vi "Create Report subVI.vi"(8 "error in (no error)":errorcluster) -> (0 "error out":errorcluster, 3 "new file path (Not A Path if cancelled)":path)   [LabVIEW 2016]
uses:
  <vilib>/Utility/sysdir.llb/System Directory Type.ctl
  <vilib>/Utility/file.llb/Write Delimited Spreadsheet (DBL).vi
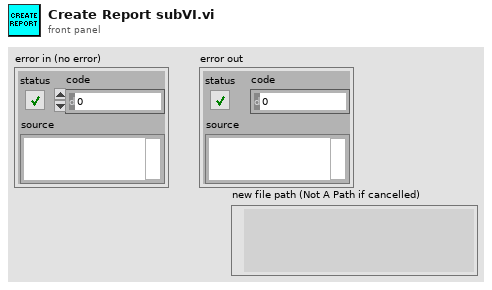
[diagram p1: front panel]
types:
  T1 = typedef "System Directory Type.ctl" = i32
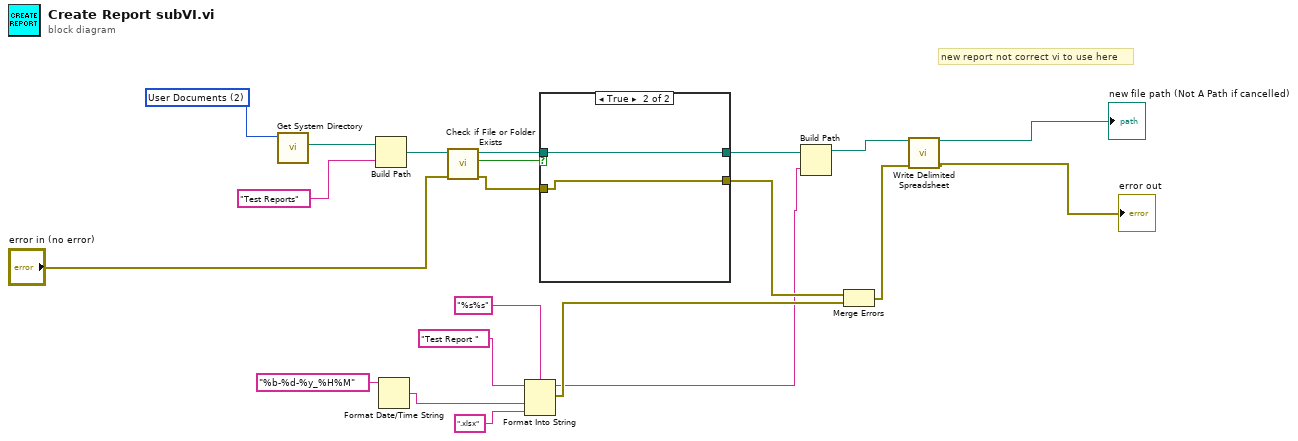
[diagram p0: block diagram]
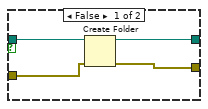
[diagram p2: hidden frame]
diagram:
  w6 = T1 2 items=["User Home"=0, "User Desktop"=1, "User Documents"=2, "User Application Data"=3, "User Preferences"=4, "User Temporary"=5, "Public Documents"=6, "Public Application Data"=7, "Public Preferences"=8, "Public Cache"=13, "System Core Libraries"=9, "System Installed Libraries"=10, "Application Files"=11, "Boot Volume Root"=12] ("system directory type")
  # "new report not correct vi to use here"
  n1 = call <vilib>:"Get System Directory.vi"("system directory type"=w6) -> ("system directory"=w8:path)  [unwired: 10 in]
  n2 = Build Path(base path=w8, name or relative path="Test Reports") -> (appended path=w9:path)
  n3 = Format Date/Time String(time format string (%c)="%b-%d-%y_%H%M") -> (date/time string=w16:string)  [unwired: 2 in]
  n4 = call <vilib>:"Check if File or Folder Exists.vi"("error in (no error)"="error in (no error)", "path"=w9) -> ("error out"=w13:errorcluster, "file or folder exists?"=w11:bool, "dup path"=w12:path)  [unwired: 7 in]
  n5 = Format Into String(format string="%s%s", initial string="Test Report ", w16, ".xlsx") -> (resulting string=w5:string, error out=w17:errorcluster)  [unwired: 1 in]
  n6 = case shown="True" w11 {
    tunnel: w12 -> [w25 w27]
    tunnel: w13 -> [w24 w26]
    tunnel: [w23 w27] -> w14
    tunnel: [w22 w26] -> w18
    frame False {
      n7 = Create Folder(path (use dialog)=w25, error in=w24) -> (created path=w23:path, error out=w22:errorcluster)  [unwired: 1 in, 1 out]
    }
    frame True {
    }
  }
  n8 = Build Path(base path=w14, name or relative path=w5) -> (appended path=w4:path)
  n9 = Merge Errors(w18, w17) -> (w2:errorcluster)
  n10 = call-poly <vilib>:"Write Delimited Spreadsheet.vi"("file path (dialog if empty)"=w4, "error in (no error)"=w2) -> ("new file path (Not A Path if cancelled)"=→"new file path (Not A Path if cancelled)":path, "error out"=→"error out":errorcluster)  [unwired: 12 in]
